vi "TS Status.vi"(8 "error in (no error)":errorcluster, 11 "Test Stand in":refnum<class "Cryo Sep Test Stand.lvclass">) -> (0 "error out":errorcluster, 3 "Test Stand out":refnum<class "Cryo Sep Test Stand.lvclass">)   [LabVIEW 2019, in "Test Stands.lvlib" / "Cryo Sep Test Stand.lvclass"]
uses:
  Cryo Sep Test Stand.lvclass
  Results/Results Method.ctl
  Results/Results.lvlib
  Generic Test Stand/Generic Test Stand.lvclass
  C:/Users/wg/Documents/LV_Projects/test-stand/App/Generic Test Stand/Generic Test Stand.lvclass
  Results/Cryo Sep Results/Cryo Sep Results.lvclass
  C:/Users/wg/Documents/LV_Projects/test-stand/App/Results/Results.lvclass
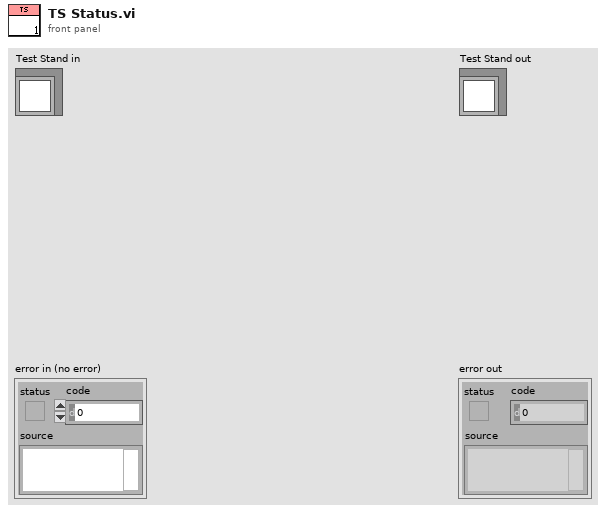
[diagram p1: front panel]
types:
  T1 = typedef "Results.lvlib/Results Method.ctl" = enum16{"Get", "Set"}
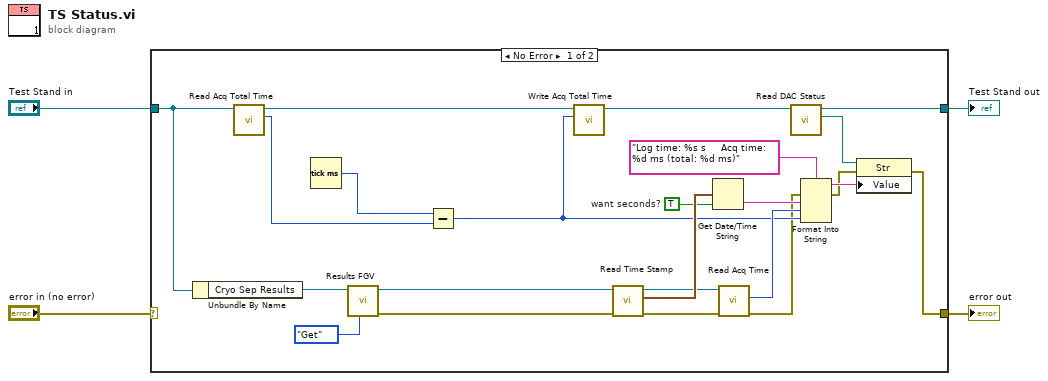
[diagram p0: block diagram]
diagram:
  n1 = case shown="No Error" "error in (no error)" {
    selector: "error in (no error)" -> [_ w29]
    tunnel: [w16 w29] -> w1
    tunnel: [w20 w28] -> w2
    tunnel: "Test Stand in" -> [w15 w28]
    frame No Error {
      w22 = TRUE  # want seconds?
      n2 = Unbundle By Name(w15) -> ("Cryo Sep Results"=w27:refnum<class "Cryo Sep Results.lvclass">)
      n3 = call "Read Acq Total Time.vi"("Generic Test Stand in"=w15) -> ("Acq Total Time"=w12:u32, "Generic Test Stand out"=w14:refnum<class "Cryo Sep Test Stand.lvclass">)  [unwired: 8 in, 1 out]
      n4 = Tick Count (ms)() -> (millisecond timer value=w25:u32)
      n5 = call-dynamic "Results FGV.vi"("Method"=Results_Method."Get", "Results in"=w27) -> ("error out"=w7:errorcluster, "Results out"=w11:refnum<class "Cryo Sep Results.lvclass">)  [unwired: 8 in]
      n6 = Subtract(x=w25, y=w12) -> (x-y=w8:u32)
      n7 = call "Write Acq Total Time.vi"("Acq Total Time"=w8, "Generic Test Stand in"=w14) -> ("Generic Test Stand out"=w13:refnum<class "Cryo Sep Test Stand.lvclass">)  [unwired: 8 in, 1 out]
      n8 = call-dynamic "Read Time Stamp.vi"("error in (no error)"=w7, "Results in"=w11) -> ("error out"=w6:errorcluster, "Time Stamp"=w23:timestamp, "Results out"=w10:refnum<class "Cryo Sep Results.lvclass">)  [unwired: 7 in]
      n9 = Get Date/Time String(seconds (now)=w23, want seconds? (F)=w22) -> (time string=w21:string)  [unwired: 1 in, 1 out]
      n10 = call "Read Acq Time.vi"("error in (no error)"=w6, "Results in"=w10) -> ("error out"=w5:errorcluster, "Acq Time"=w9:u32)  [unwired: 7 in, 1 out]
      n11 = call "Read DAC Status.vi"("Generic Test Stand in"=w13) -> ("DAC Status"=w19:refnum<vi>, "Generic Test Stand out"=w20:refnum<class "Cryo Sep Test Stand.lvclass">)  [unwired: 8 in, 1 out]
      n12 = Format Into String(format string="Log time: %s s     Acq time: %d ms (total: %d ms)", error in=w5, w21, w9, w8) -> (resulting string=w18:string, error out=w17:errorcluster)  [unwired: 1 in]
      n13 = property class="Str"(reference=w19, error in=w17, "Value"=w18) -> (error out=w16:errorcluster)  [unwired: 1 out]
    }
    frame Error {
    }
  }
  "error out" <- w1
  "Test Stand out" <- w2
